vi "ThingworxAppKey.vi"() -> (3 "Device Out":T1)   [LabVIEW 2016]
uses:
  Program Files (x86)/National Instruments/LabVIEW 2017/user.lib/IoT Devices/_subVIs/Device.ctl
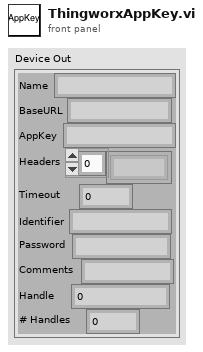
[diagram p1: front panel]
types:
  T1 = typedef "Device.ctl" = cluster{"Name":string, "BaseURL":string, "AppKey":string, "Headers":string[], "Timeout":i32, "Identifier":string, "Password":string, "Comments":string, "Handle":u32, "# Handles":i32}
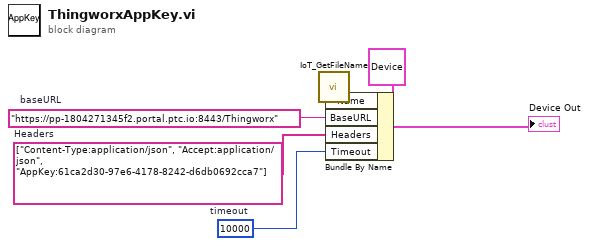
[diagram p0: block diagram]
diagram:
  w5 = string[] ["Content-Type:application/json", "Accept:application/json", "AppKey:61ca2d30-97e6-4178-8242-d6db0692cca7"]  # Headers
  w2 = 10000  # timeout
  w3 = "https://pp-1804271345f2.portal.ptc.io:8443/Thingworx"  # baseURL
  n1 = call "IoT_GetFileName.vi"() -> ("FileName"=w1:string)  [unwired: 11 in]
  n2 = Bundle By Name(cluster=T1 {"Name"="", "BaseURL"="", "AppKey"="", "Headers"=["Content-Type:application/json"], "Timeout"=10000, "Identifier"="", "Password"="", "Comments"="", "Handle"=0, "# Handles"=0} ("Device Out"), "Name"=w1, "BaseURL"=w3, "Headers"=w5, "Timeout"=w2) -> (→"Device Out":T1)
